vi "FIX_ON-OFF.vi"(8 "error in (no error)":errorcluster, 10 "Boolean":bool, 11 "channel":refnum<k24>) -> (0 "error out":errorcluster)   [LabVIEW 2021]
uses:
  F:/2PhotonVision/psychometric_function_v2/lib/Grpc.Core.dll
  lib/Grpc.Core.dll
  F:/2PhotonVision/psychometric_function_v2/lib/FossilProtosSharp.dll
  lib/FossilProtosSharp.dll
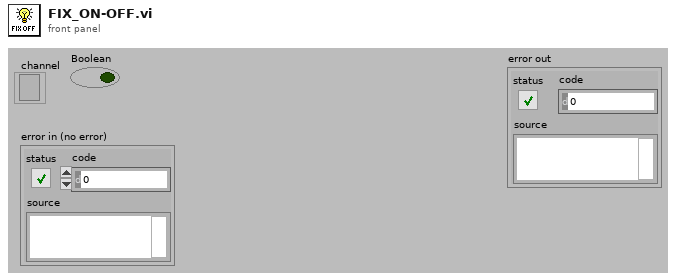
[diagram p1: front panel]
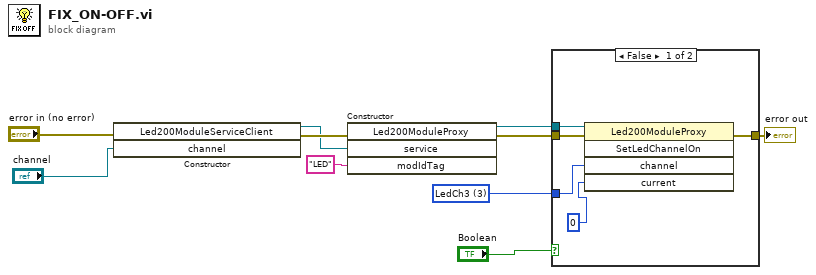
[diagram p0: block diagram]
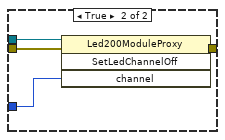
[diagram p2: hidden frame]
diagram:
  w10 = 3 items=["LedChUnspecified", "LedCh1", "LedCh2", "LedCh3", "LedCh4"] ("channel")
  n1 = constructor class="Led200ModuleServiceClient"(error in="error in (no error)", "channel"="channel") -> (reference out=w6:refnum<k24>, error out=w7:errorcluster)  [unwired: 2 in, 2 out]
  n2 = constructor class="Led200ModuleProxy"(error in=w7, "service"=w6, "modIdTag"="LED") -> (reference out=w3:refnum<k24>, error out=w2:errorcluster)  [unwired: 2 in, 3 out]
  n3 = case shown="False" "Boolean" {
    tunnel: w10 -> [w13 w19]
    tunnel: [w12 w18] -> w8
    tunnel: w3 -> [w15 w17]
    tunnel: w2 -> [w14 w16]
    frame False {
      n4 = invoke class="Led200ModuleProxy" method="SetLedChannelOn"(reference=w15, error in=w14, "channel"=w13, "current"=0) -> (error out=w12:errorcluster)  [unwired: 1 in, 4 out]
    }
    frame True {
      n5 = invoke class="Led200ModuleProxy" method="SetLedChannelOff"(reference=w17, error in=w16, "channel"=w19) -> (error out=w18:errorcluster)  [unwired: 1 in, 3 out]
    }
  }
  "error out" <- w8
